vi "BL_GetLibVersion.vi"(8 "error in (no error)":errorcluster, 11 "Potentiostat Galvanostat in":refnum<class "Potentiostat Galvanostat.lvclass">) -> (0 "error out":errorcluster, 2 "Version":string, 3 "Potentiostat Galvanostat out":refnum<class "Potentiostat Galvanostat.lvclass">)   [LabVIEW 2018, in "Potentiostat Galvanostat.lvclass"]
uses:
  Potentiostat Galvanostat.lvclass
  Potentiostat Galvanostat.lvclass/Potentiostat Galvanostat.ctl
  BL_GetErrorMsg.vi
  <vilib>/Utility/error.llb/Error Cluster From Error Code.vi
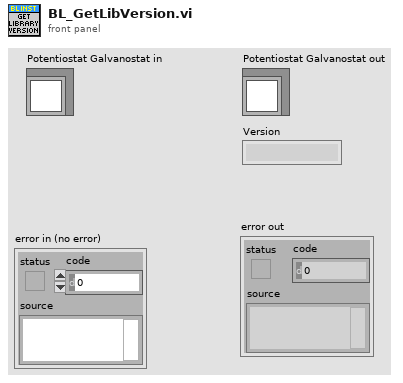
[diagram p1: front panel]
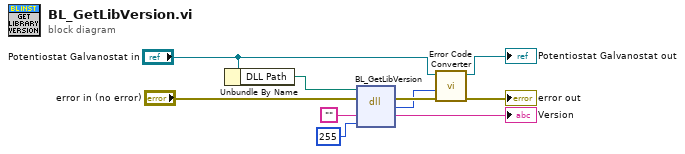
[diagram p0: block diagram]
diagram:
  n1 = Unbundle By Name("Potentiostat Galvanostat in") -> ("DLL Path"=w3:path)
  n2 = dll-call lib="C:/Projects/LabVIEW/BioLogic Instrument Driver/libs/EC-Lab Development Package/EClib.*" fn="BL_GetLibVersion"(path in=w3, error in="error in (no error)", "Version"="", "Size"=u32 255 ("StringMaxLength")) -> (error out=w4:errorcluster, "Error Code"=w2:i32, "Version"=→"Version":string)  [unwired: 2 in, 1 out]
  n3 = call "Error Code Converter.vi"("error in (no error)"=w4, "Error Code"=w2, "Potentiostat Galvanostat in"="Potentiostat Galvanostat in") -> ("error out"=→"error out":errorcluster, "Potentiostat Galvanostat out"=→"Potentiostat Galvanostat out":refnum<class "Potentiostat Galvanostat.lvclass">)  [unwired: 7 in]
